vi "Build Transfer Group.vi"(8 "error in (no error)":errorcluster, 10 "Transfer Group in":refnum<class "Transfer Group.lvclass">, 11 "Transceiver Thread in":refnum<class "Transceiver Thread.lvclass">) -> (0 "error out":errorcluster, 2 "Transfer Group out":refnum<class "Transfer Group.lvclass">, 3 "Transceiver Thread out":refnum<class "Transceiver Thread.lvclass">)   [LabVIEW 2017, in "Data Sharing Framework Core.lvlib" / "Data Sharing Framework Engine.lvlib" / "Transceiver Thread.lvclass"]
uses:
  Transceiver Thread.lvclass
  Transfer Group/Transfer Group.lvclass
  Transfer Group/Transfer Group.lvclass/Transfer Group.ctl
  Transfer/Transfer.lvclass/Transfer.ctl
  Transceiver Thread.lvclass/Transceiver Thread.ctl
  Memory/Double Pointer/Double Pointer.lvclass/Double Pointer.ctl
  <vilib>/National Instruments/Memory Manager/Classes/Pointer/Memory.Pointer.lvclass/Memory.Pointer.ctl
  Memory/Memory Buffer/Insert Channels and Preserve Value.vi
  Transfer/Get String Buffer.vi
  Transfer/Get Intermediate Buffer.vi
  Set Channels Buffer.vi
  Get Channels Buffer.vi
  Transfer/Get Channel Blocks.vi
  Memory/Double Pointer/Read Double Pointer.vi
  Memory/Double Pointer/Get Channel Count.vi
  <vilib>/National Instruments/Memory Manager/Classes/Pointer/Memory.Pointer.Read.vi
  <vilib>/National Instruments/Memory Manager/Classes/Pointer/Memory.Pointer.Read.1D.DBL.vi
  <vilib>/National Instruments/Memory Manager/Classes/Pointer/Memory.Pointer.Read.No Check.1D.DBL.vi
  <vilib>/National Instruments/Memory Manager/Classes/Pointer/Memory.Pointer.Parameter Check.Null Pointer.vi
  <vilib>/National Instruments/Memory Manager/Classes/Pointer/Memory.Pointer.Parameter Check.Subset.Power of 2.vi
  <vilib>/National Instruments/Memory Manager/Classes/Pointer/Memory.Pointer.Get Address.vi
  <vilib>/National Instruments/Memory Manager/Classes/Pointer/Memory.Pointer.Errors.vi
  <vilib>/National Instruments/Memory Manager/Classes/Pointer/Memory.Pointer.Errors.Null Pointer.vi
  <vilib>/National Instruments/Memory Manager/Classes/Pointer/Memory.Pointer.Errors.Out of Bounds.vi
  <vilib>/National Instruments/Memory Manager/Classes/Pointer/Memory.Pointer.Get Size.vi
  <vilib>/National Instruments/Memory Manager/Classes/Pointer/Memory.Pointer.Count to Size.Power of 2.vi
  <vilib>/National Instruments/Memory Manager/Classes/Pointer/Memory.Pointer.Errors.Create Error.vi
  <vilib>/NI/Static Error Handling/VIs/Static Error Handling.Source Buffer.Write.String.vi
  <vilib>/National Instruments/Memory Manager/Classes/Pointer/Memory.Pointer.Errors.Write Pointer Size.vi
  <vilib>/NI/Static Error Handling/VIs/Static Error Handling.Source Buffer.Write.Numeric.Scalar.Base10.vi
  <vilib>/NI/Static Error Handling/VIs/Static Error Handling.Source Buffer.Write.Numeric.Scalar.Base10 (U64).vi
  <vilib>/NI/Static Error Handling/VIs/Static Error Handling.Error Cluster Constant.vi
  <vilib>/NI/Static Error Handling/VIs/Static Error Handling.Error Cluster Constant (512B).vi
  <vilib>/NI/Static Error Handling/VIs/Static Error Handling.Parameters.Status.Set.vi
  <vilib>/NI/Static Error Handling/VIs/Static Error Handling.Parameters.Code.Set.vi
  <vilib>/NI/Static Error Handling/VIs/Static Error Handling.Parameters.VI Source.Set.vi
  <vilib>/National Instruments/Memory Manager/Constants/Memory.Constants.vi
  <vilib>/National Instruments/Memory Manager/Constants/Memory.Constants.Library Name.vi
  <vilib>/National Instruments/Memory Manager/Classes/Pointer/Memory.Pointer.Errors.Get Info.vi
  Memory/Double Pointer/Double Pointer.lvclass
  C:/Program Files (x86)/National Instruments/LabVIEW 2017/vi.lib/National Instruments/Memory Manager/Classes/Pointer/Memory.Pointer.lvclass
  Memory/Memory Buffer/Write Memory Buffer.vi
  Memory/Memory Buffer/Write 1D Array of U64.vi
  Memory/Memory Buffer/Write 1D Array of U32.vi
  Memory/Memory Buffer/Write 1D Array of U16.vi
  Memory/Memory Buffer/Write 1D Array of U8.vi
  Memory/Memory Buffer/Write 1D Array of I64.vi
  Memory/Memory Buffer/Write 1D Array of I32.vi
  Memory/Memory Buffer/Write 1D Array of I16.vi
  Memory/Memory Buffer/Write 1D Array of I8.vi
  Memory/Memory Buffer/Write 1D Array of Double.vi
  Memory/Memory Buffer/Write 1D Array of Single.vi
  Memory/Memory Buffer/Write 1D Array of Boolean.vi
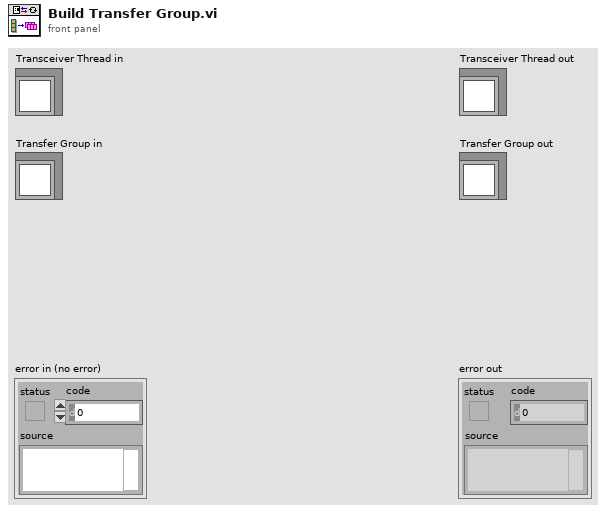
[diagram p1: front panel]
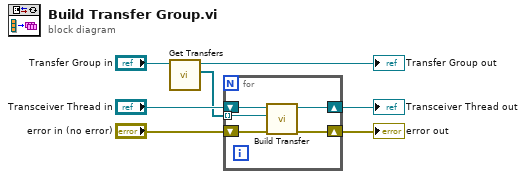
[diagram p0: block diagram]
diagram:
  n1 = call "Get Transfers.vi"("Transfer Group in"="Transfer Group in") -> ("Transfers"=w5:refnum<class "Transfer.lvclass">[], "Transfer Group out"=→"Transfer Group out":refnum<class "Transfer Group.lvclass">)  [unwired: 9 in]
  n2 = for {
    tunnel: w5 -> [w8] mode=indexing
    shift-right: [w9] -> w4
    shift-left: "Transceiver Thread in" -> [w10]
    shift-right: [w11] -> w3
    shift-left: "error in (no error)" -> [w12]
    n3 = call "Build Transfer.vi"("error in (no error)"=w12, "Transfer"=w8, "Transceiver Thread in"=w10) -> ("error out"=w11:errorcluster, "Transceiver Thread out"=w9:refnum<class "Transceiver Thread.lvclass">)  [unwired: 7 in]
  }
  "error out" <- w3
  "Transceiver Thread out" <- w4
